vi "HUSOO228.vi"() -> ()   [LabVIEW 2019]
uses:
  <vilib>/LabVIEW Interface for Arduino/Type Defs/Board Type.ctl
  <vilib>/LabVIEW Interface for Arduino/LabVIEW Interface for Arduino.lvlib
panel:
  in  "milliseconds to wait":u32
  in  "error out":errorcluster
  out "Waveform Chart":dbl(graph)
  in  "Photo Cell Pin (0)":u8
  in  "Blue Pin":u8
  in  "Green Pin":u8
  in  "Red Pin":u8
  in  "stop":bool
  in  "VISA resource":refnum<visa-resource-name>
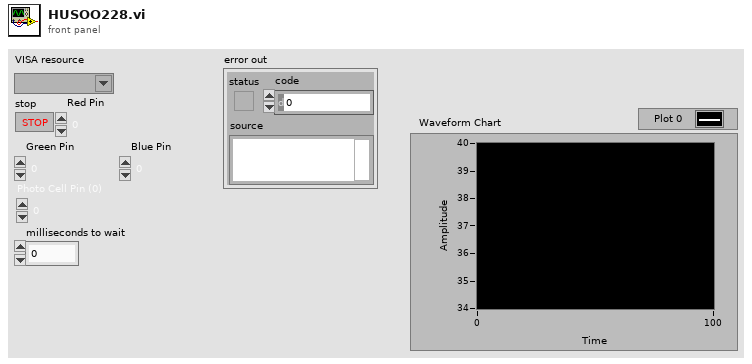
[diagram p1: front panel]
types:
  T1 = typedef "LabVIEW Interface for Arduino.lvlib/Board Type.ctl" = enum16{"Uno", "Dimuelanove w/Atmega 328", "Mega 2560"}
  T2 = typedef "LabVIEW Interface for Arduino.lvlib/Arduino Resource.ctl" = cluster{"VISA resource":refnum<visa-resource-name>, "Board Type":T1, "Connection Type":enum8{"USB / Serial"}, "Bytes Per Packet (15)":u8}
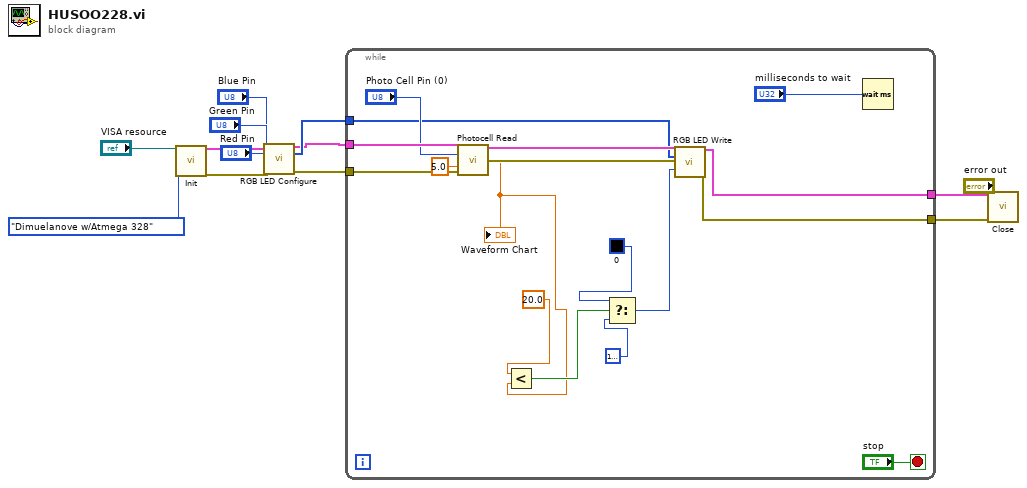
[diagram p0: block diagram]
diagram:
  n1 = call <vilib>:"Init.vi"("VISA resource"="VISA resource", "Board Type (Uno)"=Board_Type."Dimuelanove w/Atmega 328") -> ("Arduino Resource"=w10:T2, "error out"=w9:errorcluster)  [unwired: 16 in]
  n2 = call <vilib>:"RGB LED Configure.vi"("Arduino Resource"=w10, "Red Pin"="Red Pin", "Green Pin"="Green Pin", "Blue Pin"="Blue Pin", "error in"=w9) -> ("Arduino Resource"=w4:T2, "RGB LED Pins"=w5:u8[], "error out"=w3:errorcluster)  [unwired: 8 in]
  n3 = while {
    tunnel: w5 -> [w22]
    tunnel: w4 -> [w28]
    tunnel: w3 -> [w27]
    tunnel: [w21] -> w2
    tunnel: [w20] -> w1
    stop <- "stop" stop-if-true
    n4 = call <vilib>:"Photocell Read.vi"("Arduino Resource"=w28, "Photo Cell Pin (0)"="Photo Cell Pin (0)", "Vcc (5)"=5.0, "error in"=w27) -> ("Arduino Resource"=w24:T2, "Light Intensity (0 - 100)"=w16:dbl, "error out"=w23:errorcluster)  [unwired: 9 in]
    "Waveform Chart" <- w16
    n5 = Less?(x=20.0, y=w16) -> (x < y?=w18:bool)
    n6 = Select(t=u32 0 ("Color"), s=w18, f=u32 16777225 ("Color")) -> (s? t:f=w13:u32)
    n7 = call <vilib>:"RGB LED Write.vi"("Arduino Resource"=w24, "RGB LED Pins"=w22, "Color"=w13, "error in"=w23) -> ("Arduino Resource"=w21:T2, "error out"=w20:errorcluster)  [unwired: 9 in, 1 out]
    n8 = Wait (ms)(milliseconds to wait="milliseconds to wait") -> ()  [unwired: 1 out]
  }
  n9 = call <vilib>:"Close.vi"("Arduino Resource"=w2, "error in"=w1) -> ()  [unwired: 13 in, 1 out]
